vi "FPGA COUNTER AND VELOCITY.vi"() -> ()   [LabVIEW 2017]
uses:
  <vilib>/Platform/TimedLoop/XDataNode/timing_clust.ctl
  <vilib>/Platform/TimedLoop/XDataNode/nitl_modes.ctl
  <vilib>/Platform/TimedLoop/XDataNode/wakeup.ctl
  <vilib>/rvi/Emulation/niFpgaSctlEmulationGetInTimedLoop.vi
  <vilib>/rvi/Emulation/niFpgaEmulationReportErrorSimple.vi
  <vilib>/rvi/Emulation/niFpgaGetClockAttributes.vi
  <vilib>/rvi/Emulation/niFpgaCriticalErrorInLSC.vi
  <vilib>/Platform/TimedLoop/XDataNode/XDataNode.xnode
  <vilib>/Platform/TimedLoop/XDataNode/XDNodeRunTimeDep.lvlib
panel:
  out "Pulses/Millisecond":u32
  out "Pulse Value":u32
  out "*2.5E-8 Second/Period":u32
  in  "Signal":bool
  in  "Direction":bool
  in  "Reset":bool
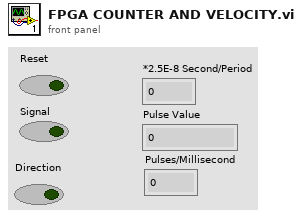
[diagram p1: front panel]
types:
  T1 = typedef "XDNodeRunTimeDep.lvlib/timing_clust.ctl" = cluster{"Expected End [f-1]":u64, "Actual End [f-1]":u64, "Finished Late? [f-1]":bool, "Expected End [i-1]":u64, "Actual End [i-1]":u64, "Finished Late? [i-1]":bool, "Expected Start [i]":u64, "Actual Start [i]":u64, "Expected Start [f]":u64, "Actual Start [f]":u64, "Source Name":string, "Structure Name":string, "Period":i64, "Deadline":i64, "Offset":i64, "Start":i64, "Priority":i32, "Timeout":i32, "Mode":T2, "Wakeup Reason":T3, "Error":errorcluster, "Source Type":string, "Secondary Source Type":string, "Global End Time":u64, "Global Start Time":u64, "Frame Duration":u64, "Iteration Duration":u64, "Assigned CPU":i32, "I/O Scan Engine Mode":u32}
  T2 = typedef "XDNodeRunTimeDep.lvlib/nitl_modes.ctl" = enum32{"No Change", "Process missed periods, maintain original phase", "Discard missed periods, maintain original phase", "Process missed periods, ignore original phase", "Discard missed periods, ignore original phase"}
  T3 = typedef "XDNodeRunTimeDep.lvlib/wakeup.ctl" = enum32{"Normal", "Aborted", "Asynchronous wakeup", "Timing source error", "Timed loop error", "Timeout"}
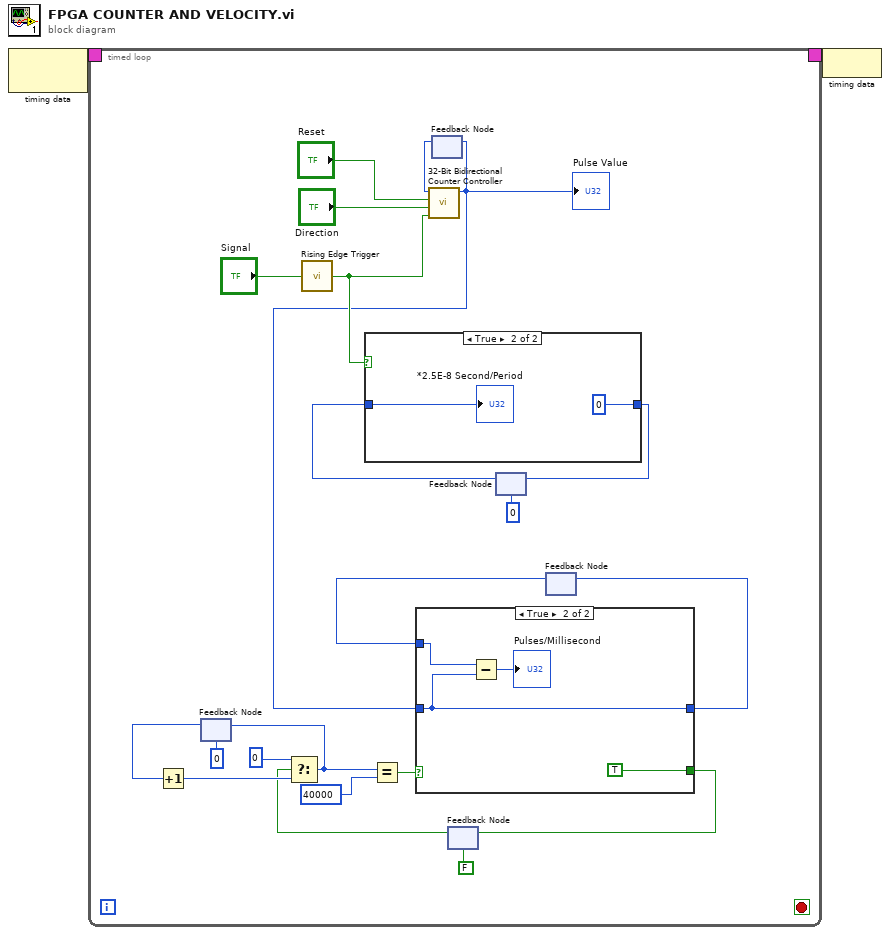
[diagram p0: block diagram]
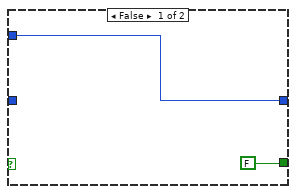
[diagram p2: hidden frame]
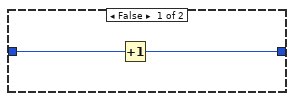
[diagram p3: hidden frame]
diagram:
  n1 = node-c288() -> (w2:T1)  [unwired: 1 in]
  n2 = timed-loop {
    timing: w2 -> [_]
    timing-out: [_] -> w1
    stop <- _ stop-if-true
    n3 = feedback #1(u32 0 ("t")) -> (w15:u32)
    n4 = Increment(x=w15) -> (x+1=w16:u32)
    n5 = call "Rising Edge Trigger.vi"("Signal"="Signal") -> ("Trigger?"=w19:bool)
    n6 = feedback #2() -> (w23:u32)  [unwired: 1 in]
    n7 = call "32-Bit Bidirectional Counter Controller.vi"("Enable"=w19, "Direction"="Direction", "Reset"="Reset", "Value"=w23) -> ("Value+"=w10:u32)  [unwired: 7 in]
    "Pulse Value" <- w10
    n8 = feedback-in #2(w10) -> ()
    n9 = feedback #3(FALSE) -> (w8:bool)
    n10 = Select(t=u32 0, s=w8, f=w16) -> (s? t:f=w14:u32)
    n11 = feedback-in #1(w14) -> ()
    n12 = Equal?(x=w14, y=u32 40000) -> (x = y?=w12:bool)
    n13 = feedback #4(i16 0) -> (w18:i16)
    n14 = case shown="True" w19 {
      tunnel: [w31 i16 0] -> w4
      tunnel: w18 -> [w30 w32]
      frame False {
        n15 = Increment(x=w30) -> (x+1=w31:i16)
      }
      frame True {
        "*2.5E-8 Second/Period" <- w32
      }
    }
    n16 = feedback-in #4(w4) -> ()
    n17 = feedback #5() -> (w5:u32)  [unwired: 1 in]
    n18 = case shown="True" w12 {
      tunnel: w10 -> [_ w27]
      tunnel: [FALSE TRUE] -> w9
      tunnel: [w24 w27] -> w6
      tunnel: w5 -> [w24 w28]
      frame False {
      }
      frame True {
        n19 = Subtract(x=w28, y=w27) -> (x-y=→"Pulses/Millisecond":u32)
      }
    }
    n20 = feedback-in #3(w9) -> ()
    n21 = feedback-in #5(w6) -> ()
  }
  n22 = node-c288(w1) -> ()
